vi "Set Subject.vi"(8 "error in (no error)":errorcluster, 10 "Subject":string, 11 "Gmail in":refnum<class "Gmail.lvclass">) -> (0 "error out":errorcluster, 3 "Gmail out":refnum<class "Gmail.lvclass">)   [LabVIEW 2020, in "Gmail API.lvlib" / "Gmail.lvclass"]
doc: "Sets the subject line for the email."
uses:
  Gmail.lvclass
  Gmail.lvclass/Gmail.ctl
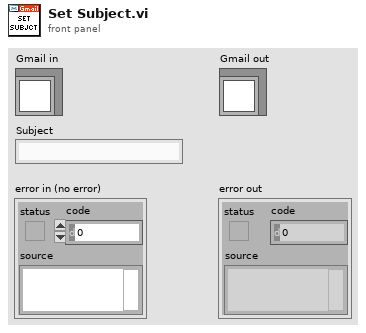
[diagram p1: front panel]
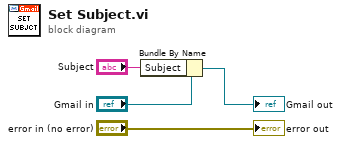
[diagram p0: block diagram]
diagram:
  n1 = Bundle By Name(cluster="Gmail in", "Subject"="Subject") -> (→"Gmail out":refnum<class "Gmail.lvclass">)
  "error out" <- "error in (no error)"
